vi "Create messenger.vi"(6 "InterComm path":path=path "../S4ICS/SubVI/S4ICS InterComm.vi", 7 "0mqComm path":path=path "../S4ICS/SubVI/S4ICS InterComm.vi", 8 "error in (no error)":errorcluster, 9 "S4statusQueueName":string, 10 "S4commandQueueName":string, 11 "Messenger in":refnum<class "Messenger.lvclass">) -> (0 "error out":errorcluster, 3 "Messenger out":refnum<class "Messenger.lvclass">)   [LabVIEW 2018, in "Messenger.lvclass"]
uses:
  Messenger.lvclass
  Messenger.lvclass/Messenger.ctl
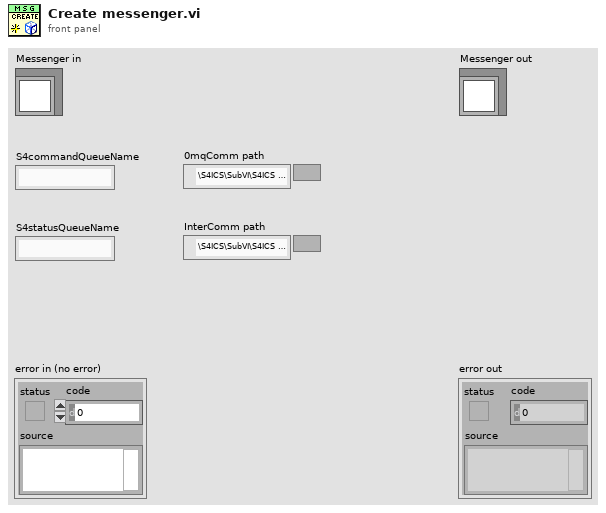
[diagram p1: front panel]
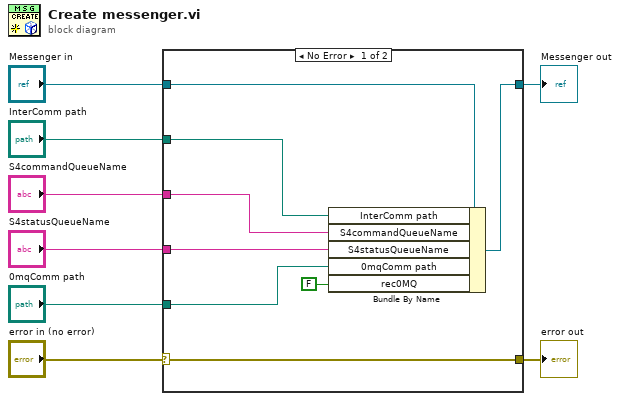
[diagram p0: block diagram]
diagram:
  n1 = case shown="No Error" "error in (no error)" {
    selector: "error in (no error)" -> [w16 w17]
    tunnel: [w16 w17] -> w7
    tunnel: [w14 w18] -> w5
    tunnel: "Messenger in" -> [w15 w18]
    tunnel: "InterComm path" -> [w13 _]
    tunnel: "S4statusQueueName" -> [w12 _]
    tunnel: "S4commandQueueName" -> [w11 _]
    tunnel: "0mqComm path" -> [w10 _]
    frame No Error {
      n2 = Bundle By Name(cluster=w15, "InterComm path"=w13, "S4commandQueueName"=w11, "S4statusQueueName"=w12, "0mqComm path"=w10, "rec0MQ"=FALSE) -> (w14:refnum<class "Messenger.lvclass">)
    }
    frame Error {
    }
  }
  "error out" <- w7
  "Messenger out" <- w5
